vi "point_frame.vi"() -> ()   [LabVIEW 2017]
uses:
  <vilib>/gmath/NI_Gmath.lvlib
panel:
  out "r 8":dbl format="%.7g"
  out "r 7":dbl format="%.7g"
  out "r 6":dbl format="%.7g"
  out "r 5":dbl format="%.7g"
  out "r 4":dbl format="%.7g"
  out "r 3":dbl format="%.7g"
  out "r 2":dbl format="%.7g"
  out "r":dbl format="%.7g"
  out "impulse szum/mean":cluster{"X":dbl, "Y":dbl}[](graph)
  in  "felharmonikus N":i32=2
  in  "SNR window width [Hz]":dbl=0.2 format="%#_13g"
  in  "Case select":string(combo)="6min"
  out "impulse mean":cluster{"X":dbl, "Y":dbl}[](graph)
  out "impulse szum":cluster{"X":dbl, "Y":dbl}[](graph)
  out "impulse sd":cluster{"X":dbl, "Y":dbl}[](graph)
  out "impulse szum/time":cluster{"X":dbl, "Y":dbl}[](graph)
  out "Menetriányú SNR (1 felharmonikus)":cluster{"X":dbl, "Y":dbl}[](graph)
  out "eredõ SNR (ugyanolyan paraméterek mint az 1.)":cluster{"X":dbl, "Y":dbl}[](graph)
  out "Menetriányú SNR (csak alapharmonikus)":cluster{"X":dbl, "Y":dbl}[](graph)
  in  "Path":path=path "C:/Users/Lenovo/Desktop/szakdoga/data/time/egyenletes_resztavok"
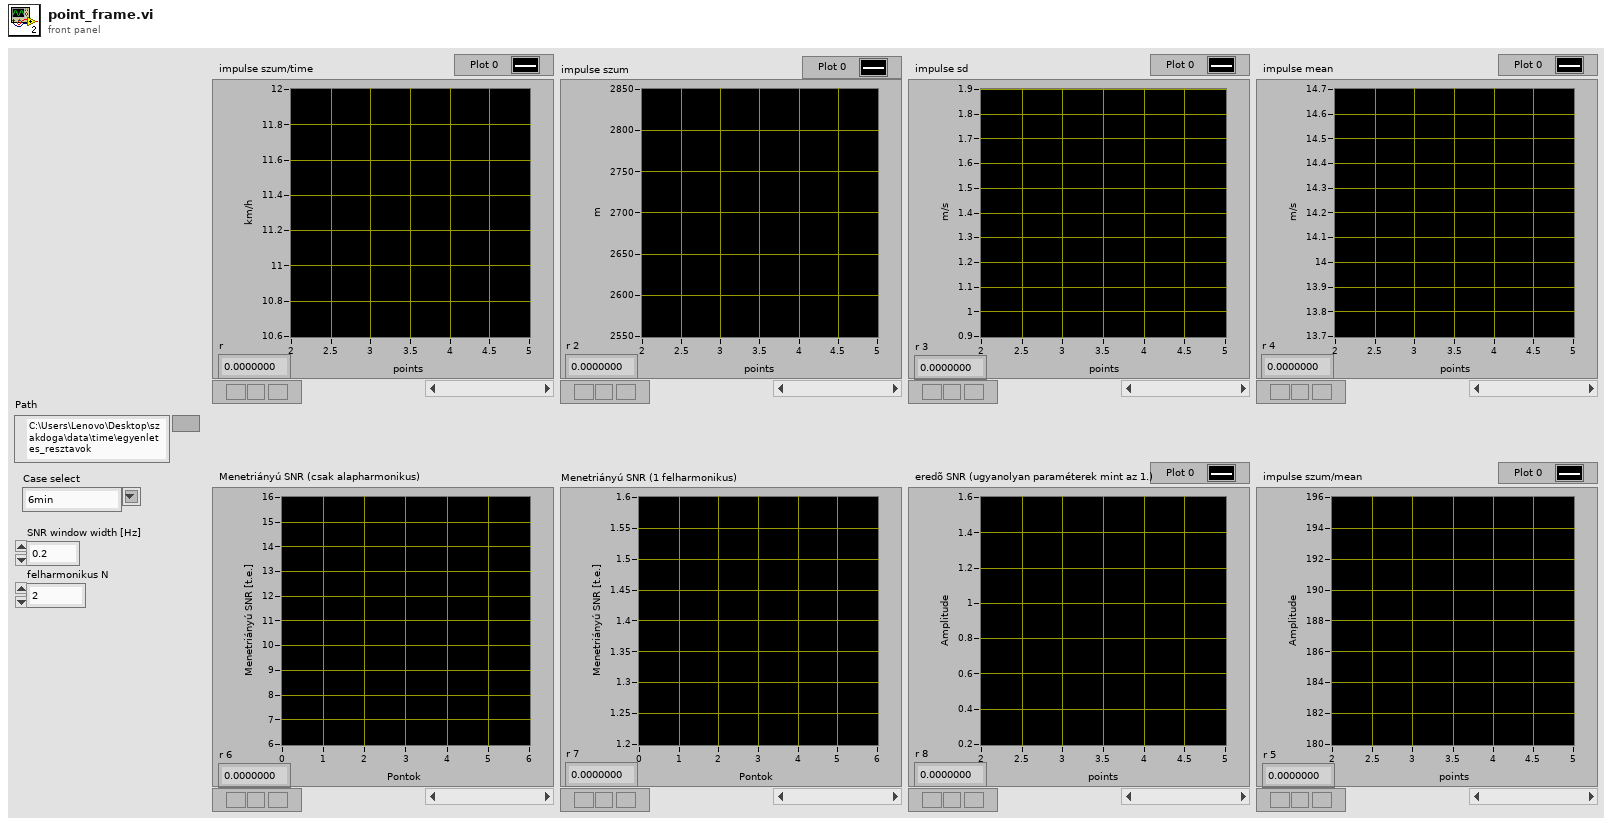
[diagram p1: front panel]
types:
  T1 = cluster{cluster{dbl, "impulse szum/time":dbl}[], cluster{dbl, "impulse  szum":dbl}[], cluster{dbl, "impulse standard deviation":dbl}[], cluster{dbl, "impulse mean":dbl}[], cluster{dbl, "X SNR 1":dbl}[], cluster{dbl, "X SNR 2":dbl}[], cluster{dbl, "X SNR 3":dbl}[], cluster{dbl, "impulse szum/avg":dbl}[]}
  T2 = cluster{cluster{dbl, dbl}[], cluster{dbl, "impulse  szum":dbl}[], cluster{dbl, "impulse standard deviation":dbl}[], cluster{dbl, "impulse mean":dbl}[], cluster{dbl, dbl}[], cluster{dbl, dbl}[], cluster{dbl, dbl}[], cluster{dbl, "impulse szum/mean":dbl}[]}
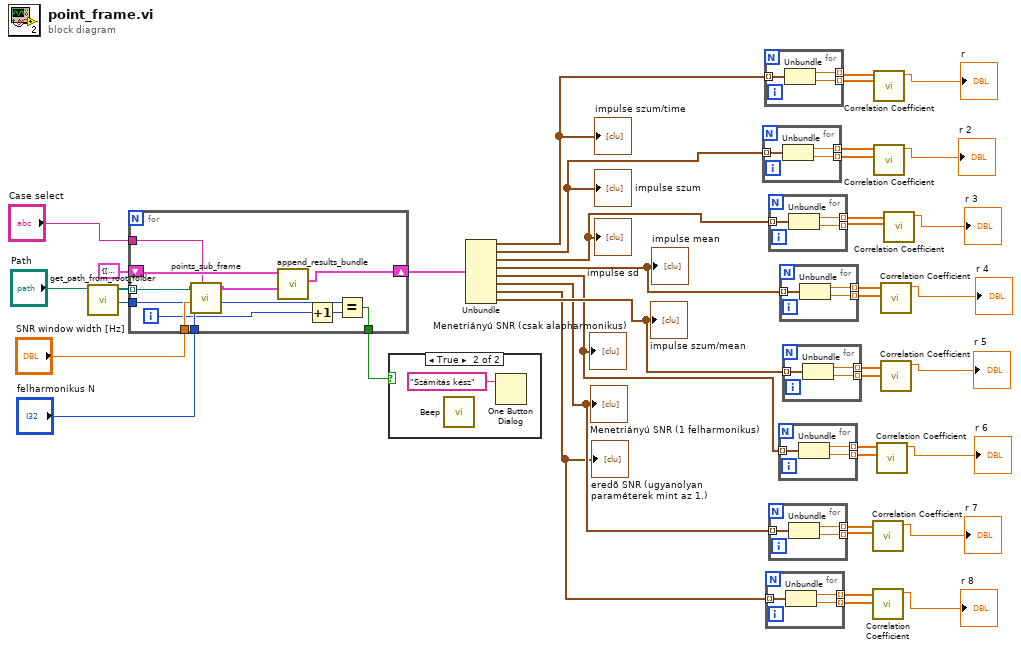
[diagram p0: block diagram]
diagram:
  n1 = call "get_path_from_root_folder.vi"("Path"="Path") -> ("Number of Files"=w36:i32, "Array"=w41:path[])  [unwired: 9 in]
  n2 = for {
    tunnel: w41 -> [w50] mode=indexing
    tunnel: "Case select" -> [w48]
    tunnel: "SNR window width [Hz]" -> [w47]
    tunnel: "felharmonikus N" -> [w46]
    tunnel: w36 -> [w45]
    tunnel: [w42] -> w35
    shift-right: [w51] -> w33
    shift-left: T1 {[], [], [], [], [], [], [], []} ("concat(X,Y)") -> [w52]
    i -> [w43]
    n3 = call "points_sub_frame.vi"("Case select"=w48, "felharmonikus N"=w46, "SNR window width [Hz]"=w47, "path to binary file"=w50) -> ("output cluster"=w49:T2)  [unwired: 7 in]
    n4 = call "append_results_bundle.vi"("Y"=w49, "X"=w52) -> ("concat(X,Y)"=w51:T1)  [unwired: 8 in]
    n5 = Increment(x=w43) -> (x+1=w44:i32)
    n6 = Equal?(x=w45, y=w44) -> (x = y?=w42:bool)
  }
  n7 = case shown="True" w35 {
    frame False {
    }
    frame True {
      n8 = call <vilib>:"Beep.vi"() -> ()  [unwired: 12 in]
      n9 = One Button Dialog(message="Számítás kész") -> ()  [unwired: 1 in, 1 out]
    }
  }
  n10 = Unbundle(w33) -> (w32:cluster{dbl, "impulse szum/time":dbl}[], w31:cluster{dbl, "impulse  szum":dbl}[], w30:cluster{dbl, "impulse standard deviation":dbl}[], w29:cluster{dbl, "impulse mean":dbl}[], w27:cluster{dbl, "X SNR 1":dbl}[], w26:cluster{dbl, "X SNR 2":dbl}[], w25:cluster{dbl, "X SNR 3":dbl}[], w28:cluster{dbl, "impulse szum/avg":dbl}[])
  "Menetriányú SNR (csak alapharmonikus)" <- w27
  "eredõ SNR (ugyanolyan paraméterek mint az 1.)" <- w25
  "Menetriányú SNR (1 felharmonikus)" <- w26
  "impulse szum/time" <- w32
  "impulse sd" <- w30
  "impulse szum" <- w31
  "impulse mean" <- w29
  "impulse szum/mean" <- w28
  n11 = for {
    tunnel: w31 -> [w56] mode=indexing
    tunnel: [w55] -> w18 mode=indexing
    tunnel: [w54] -> w17 mode=indexing
    n12 = Unbundle(w56) -> (w55:dbl, "impulse  szum"=w54:dbl)
  }
  n13 = for {
    tunnel: w32 -> [w59] mode=indexing
    tunnel: [w58] -> w24 mode=indexing
    tunnel: [w57] -> w23 mode=indexing
    n14 = Unbundle(w59) -> (w58:dbl, "impulse szum/time"=w57:dbl)
  }
  n15 = for {
    tunnel: w25 -> [w62] mode=indexing
    tunnel: [w61] -> w19 mode=indexing
    tunnel: [w60] -> w1 mode=indexing
    n16 = Unbundle(w62) -> (w61:dbl, "X SNR 3"=w60:dbl)
  }
  n17 = for {
    tunnel: w30 -> [w65] mode=indexing
    tunnel: [w64] -> w9 mode=indexing
    tunnel: [w63] -> w8 mode=indexing
    n18 = Unbundle(w65) -> (w64:dbl, "impulse standard deviation"=w63:dbl)
  }
  n19 = for {
    tunnel: w26 -> [w68] mode=indexing
    tunnel: [w67] -> w3 mode=indexing
    tunnel: [w66] -> w2 mode=indexing
    n20 = Unbundle(w68) -> (w67:dbl, "X SNR 2"=w66:dbl)
  }
  n21 = for {
    tunnel: w27 -> [w71] mode=indexing
    tunnel: [w70] -> w5 mode=indexing
    tunnel: [w69] -> w4 mode=indexing
    n22 = Unbundle(w71) -> (w70:dbl, "X SNR 1"=w69:dbl)
  }
  n23 = for {
    tunnel: w29 -> [w74] mode=indexing
    tunnel: [w73] -> w21 mode=indexing
    tunnel: [w72] -> w7 mode=indexing
    n24 = Unbundle(w74) -> (w73:dbl, "impulse mean"=w72:dbl)
  }
  n25 = for {
    tunnel: w28 -> [w77] mode=indexing
    tunnel: [w76] -> w20 mode=indexing
    tunnel: [w75] -> w6 mode=indexing
    n26 = Unbundle(w77) -> (w76:dbl, "impulse szum/avg"=w75:dbl)
  }
  n27 = call <vilib>:"Correlation Coefficient.vi"("Y"=w2, "X"=w3) -> ("correlation coefficient r"=→"r 7":dbl)  [unwired: 8 in, 1 out]
  n28 = call <vilib>:"Correlation Coefficient.vi"("Y"=w1, "X"=w19) -> ("correlation coefficient r"=→"r 8":dbl)  [unwired: 8 in, 1 out]
  n29 = call <vilib>:"Correlation Coefficient.vi"("Y"=w23, "X"=w24) -> ("correlation coefficient r"=→"r":dbl)  [unwired: 8 in, 1 out]
  n30 = call <vilib>:"Correlation Coefficient.vi"("Y"=w17, "X"=w18) -> ("correlation coefficient r"=→"r 2":dbl)  [unwired: 8 in, 1 out]
  n31 = call <vilib>:"Correlation Coefficient.vi"("Y"=w4, "X"=w5) -> ("correlation coefficient r"=→"r 6":dbl)  [unwired: 8 in, 1 out]
  n32 = call <vilib>:"Correlation Coefficient.vi"("Y"=w7, "X"=w21) -> ("correlation coefficient r"=→"r 4":dbl)  [unwired: 8 in, 1 out]
  n33 = call <vilib>:"Correlation Coefficient.vi"("Y"=w6, "X"=w20) -> ("correlation coefficient r"=→"r 5":dbl)  [unwired: 8 in, 1 out]
  n34 = call <vilib>:"Correlation Coefficient.vi"("Y"=w8, "X"=w9) -> ("correlation coefficient r"=→"r 3":dbl)  [unwired: 8 in, 1 out]
